vi "Subscribe.vi"(8 "error in (no error)":errorcluster, 10 "Subscription Request":refnum<class "SubscriptionRequest.lvclass">, 11 "Mediator In":refnum<class "Mediator.lvclass">) -> (0 "error out":errorcluster, 3 "Mediator Out":refnum<class "Mediator.lvclass">)   [LabVIEW 2015, in "Mediator.lvlib" / "Mediator.lvclass"]
uses:
  Mediator.lvclass
  IMediator/SubscriptionRequest/SubscriptionRequest.lvclass
  Mediator.lvclass/Mediator.ctl
  Topic Messages/Add Topic Subscriber Msg/Add Topic Subscriber Msg.lvclass/Add Topic Subscriber Msg.ctl
  <vilib>/ActorFramework/Message Enqueuer/Message Enqueuer.lvclass/Message Enqueuer.ctl
  <vilib>/ActorFramework/Message Enqueuer/Enqueue.vi
  <vilib>/ActorFramework/Message Priority Queue/Priority Enqueue.vi
  Topic Messages/Add Topic Subscriber Msg/Add Topic Subscriber Msg.lvclass
  TopicLookupTable/TopicLookupTable.lvclass
  Topic/Topic.lvclass
  <vilib>/ActorFramework/Actor/Actor.lvclass
panel:
  # "Who wants it?\nWhat do they want?\nWhat type are they expecting?\nHow do they want it sent?"
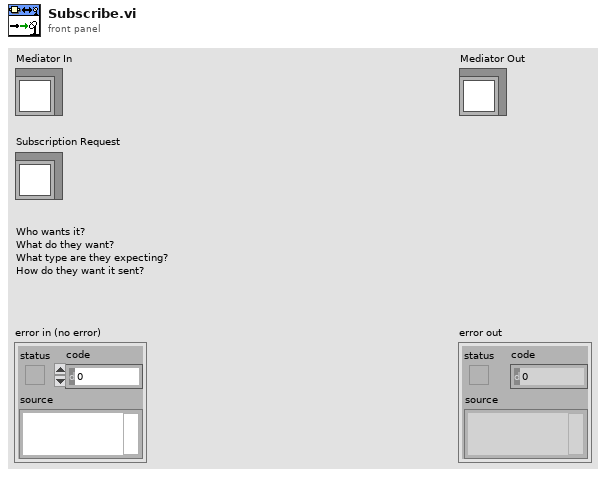
[diagram p1: front panel]
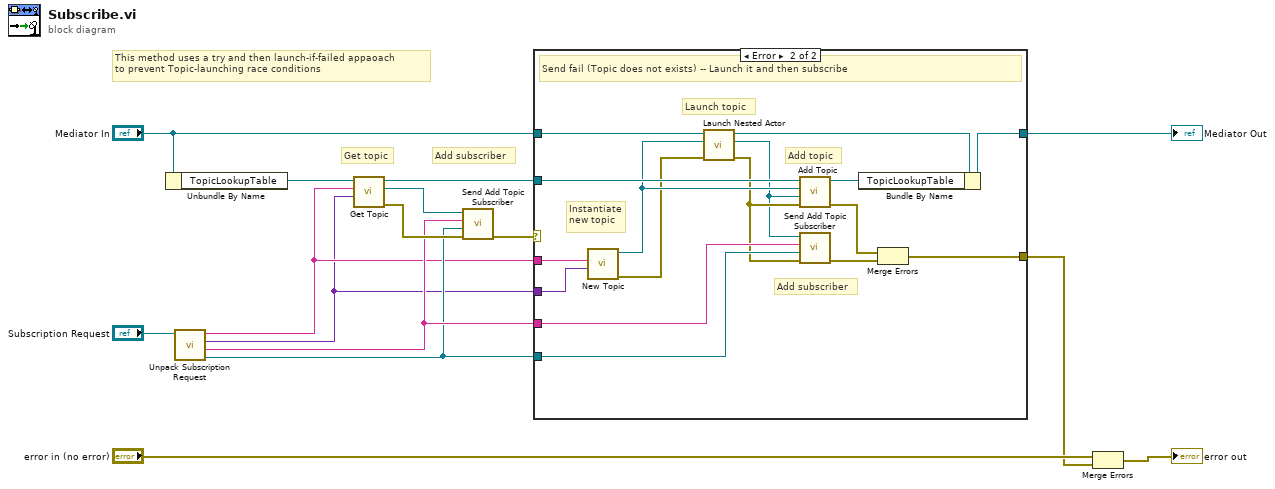
[diagram p0: block diagram]
diagram:
  # "This method uses a try and then launch-if-failed appaoach\nto prevent Topic-launching race conditions"
  # "Add subscriber"
  # "Get topic"
  n1 = Unbundle By Name("Mediator In") -> ("TopicLookupTable"=w12:refnum<class "TopicLookupTable.lvclass">)
  n2 = call "Unpack Subscription Request.vi"("SubscriptionRequest in"="Subscription Request") -> ("Transport"=w3:refnum<class "ITransport.lvclass">, "Unique Subscriber ID"=w4:string, "Type"=w1:variant, "Topic Name"=w2:string)  [unwired: 7 in]
  n3 = call "Get Topic.vi"("Topic Type"=w1, "Topic Name"=w2, "TopicLookupTable in"=w12) -> ("error out"=w6:errorcluster, "Topic Refnum"=w13:refnum<class "Message Enqueuer.lvclass">, "TopicLookupTable out"=w11:refnum<class "TopicLookupTable.lvclass">)  [unwired: 5 in, 1 out]
  n4 = call "Send Add Topic Subscriber.vi"("error in (no error)"=w6, "Subscriber Transport"=w3, "Subscriber Name"=w4, "Message Enqueuer"=w13) -> ("error out"=w8:errorcluster)  [unwired: 6 in, 1 out]
  n5 = case shown="Error" w8 {
    selector: w8 -> [w16 _]
    tunnel: w11 -> [_ w28]
    tunnel: "Mediator In" -> [w17 w33]
    tunnel: [w17 w32] -> w9
    tunnel: w2 -> [_ w30]
    tunnel: w1 -> [_ w29]
    tunnel: [w16 w20] -> w7
    tunnel: w4 -> [_ w24]
    tunnel: w3 -> [_ w23]
    frame No Error {
      # "Subscribe OK (Topic is alive)"
    }
    frame Error {
      # "Launch topic"
      # "Add topic"
      # "Add subscriber"
      # "Instantiate\nnew topic"
      # "Send fail (Topic does not exists) -- Launch it and then subscribe"
      n6 = call "New Topic.vi"("Data Type"=w29, "Name"=w30) -> ("error out"=w25:errorcluster, "Topic out"=w26:refnum<class "Topic.lvclass">)  [unwired: 8 in]
      n7 = call <vilib>:"Launch Nested Actor.vi"("error in (no error)"=w25, "Nested Actor"=w26, "Caller Actor in"=w33) -> ("error out"=w19:errorcluster, "Nested Actor's Enqueuer"=w18:refnum<class "Message Enqueuer.lvclass">, "Caller Actor out"=w31:refnum<class "Mediator.lvclass">)  [unwired: 6 in]
      n8 = call "Add Topic.vi"("error in (no error)"=w19, "Topic Enqueuer"=w18, "Topic Object"=w26, "TopicLookupTable in"=w28) -> ("error out"=w22:errorcluster, "TopicLookupTable out"=w27:refnum<class "TopicLookupTable.lvclass">)  [unwired: 5 in, 1 out]
      n9 = call "Send Add Topic Subscriber.vi"("error in (no error)"=w19, "Subscriber Transport"=w23, "Subscriber Name"=w24, "Message Enqueuer"=w18) -> ("error out"=w21:errorcluster)  [unwired: 6 in, 1 out]
      n10 = Bundle By Name(cluster=w31, "TopicLookupTable"=w27) -> (w32:refnum<class "Mediator.lvclass">)
      n11 = Merge Errors(w22, w21) -> (w20:errorcluster)
    }
  }
  "Mediator Out" <- w9
  n12 = Merge Errors("error in (no error)", w7) -> (→"error out":errorcluster)
